vi "Intan_AmpInfo.vi"(3 "error in":errorcluster, 4 "byte count":u32=500, 5 "VISA resource name":refnum<visa-resource-name>) -> (0 "error out":errorcluster, 1 "Text response":string, 2 "VISA resource name out":refnum<visa-resource-name>)   [LabVIEW 2015]
doc: "This VI queries the Intan RHD2000 chip for revision history, die revision, and number amplifiers."
panel:
  out "return count":u32
  in  "Teensy event char":string="i"
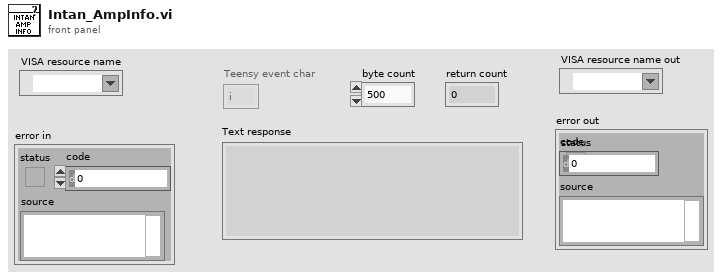
[diagram p1: front panel]
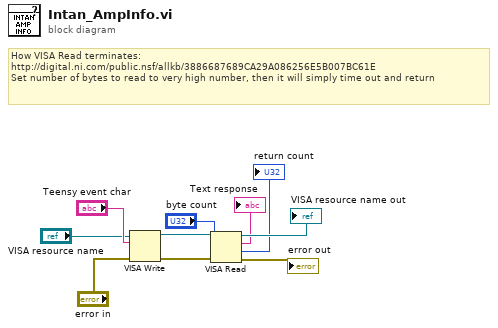
[diagram p0: block diagram]
diagram:
  # "How VISA Read terminates:\nhttp://digital.ni.com/public.nsf/allkb/3886687689CA29A086256E5B007BC61E\nSet number of bytes to read to very high number, then it will simply time out and return"
  n1 = VISA Write(VISA resource name="VISA resource name", write buffer="Teensy event char", error in (no error)="error in") -> (VISA resource name out=w5:refnum<visa-resource-name>, error out=w4:errorcluster)  [unwired: 1 out]
  n2 = VISA Read(VISA resource name=w5, byte count="byte count", error in (no error)=w4) -> (VISA resource name out=→"VISA resource name out":refnum<visa-resource-name>, read buffer=→"Text response":string, return count=→"return count":u32, error out=→"error out":errorcluster)
